vi "例程05-数据类型.vi"() -> ()   [LabVIEW 2016]
panel:
  out "date/time string":string
  out "concatenated string 2":string
  out "concatenated string":string
  out "Numeric":dbl
  in  "String":string
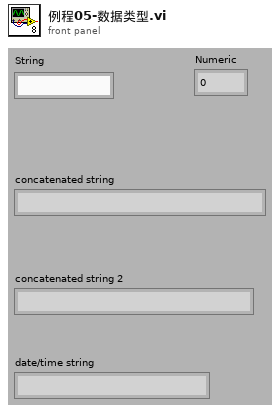
[diagram p1: front panel]
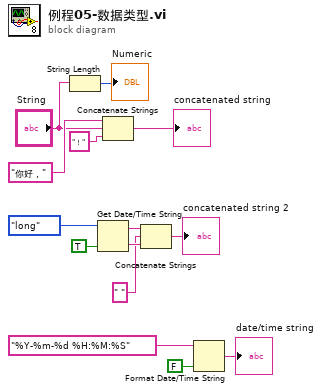
[diagram p0: block diagram]
diagram:
  n1 = String Length(string="String") -> (length=→"Numeric":i32)
  n2 = Get Date/Time String(date format (0)=enum16{"short", "long", "abbreviated"}."long", want seconds? (F)=TRUE) -> (date string=w9:string, time string=w7:string)  [unwired: 1 in]
  n3 = Concatenate Strings("你好，" ("string"), "String", "！" ("string")) -> (→"concatenated string":string)
  n4 = Concatenate Strings(w9, " " ("string"), w7) -> (→"concatenated string 2":string)
  n5 = Format Date/Time String(time format string (%c)="%Y-%m-%d %H:%M:%S", UTC format=FALSE) -> (date/time string=→"date/time string":string)  [unwired: 1 in]
